vi "enumerateStaticDependencies.vi"(8 "error in (no error)":errorcluster, 11 "SMO.A":refnum<class "SMO.ErrorInjection.lvclass">) -> (0 "error out":errorcluster, 2 "Static Dependencies":refnum<class "Dependency.lvclass">[](array[class]), 3 "SMO.A out":refnum<class "SMO.ErrorInjection.lvclass">)   [LabVIEW 2021, in "SMO.ErrorInjection.lvclass"]
uses:
  SMO.ErrorInjection.lvclass
  SMO.ErrorInjection.lvclass/SMO.ErrorInjection.ctl
  src/SMO/SMO.lvclass
  src/Dependency/Dependency.lvclass
panel:
  # "For instructions on how to use the JKI State Machine Objects, examples and video tutorials, visit:\nhttp://jki.net/state-machine-objects/\n\nJKI State Machine Objects™\nhttp://jki.net/state-machine-objects/\nCopyright (C) 2005-2015, JKI <info@jki.net>\nALL RIGHTS RESERVED"
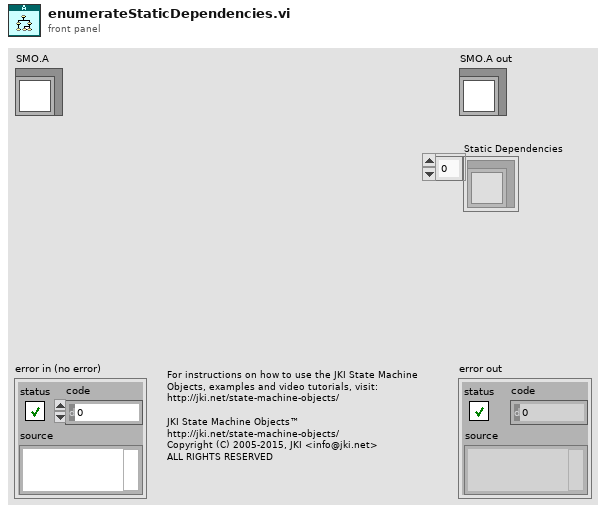
[diagram p1: front panel]
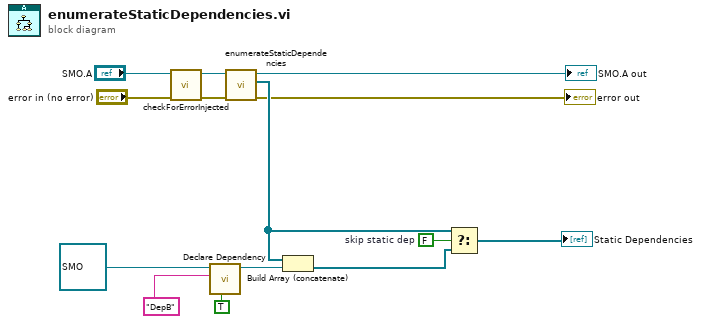
[diagram p0: block diagram]
diagram:
  w14 = FALSE  # skip static dep
  n1 = call "checkForErrorInjected.vi"("error in (no error)"="error in (no error)", "SMO.ErrorInjection in"="SMO.A") -> ("error out"=w9:errorcluster, "SMO.ErrorInjection dup"=w7:refnum<class "SMO.ErrorInjection.lvclass">)  [unwired: 8 in]
  n2 = call "Declare Dependency.vi"("Shared Resource (F)"=TRUE, "Name"="DepB", "Type"=refnum<class "SMO.lvclass"> refnum ("smo.lvlib:SMO.lvclass")) -> ("Dependency out"=w3:refnum<class "Dependency.lvclass">)  [unwired: 7 in, 1 out]
  n3 = call-parent "enumerateStaticDependencies.vi"("error in (no error)"=w9, "SMO"=w7) -> ("error out"=→"error out":errorcluster, "Static Dependencies"=w12:refnum<class "Dependency.lvclass">[], "SMO out"=→"SMO.A out":refnum<class "SMO.ErrorInjection.lvclass">)  [unwired: 7 in]
  n4 = Build Array (concatenate)(w12, w3) -> (w13:refnum<class "Dependency.lvclass">[])
  n5 = Select(t=w12, s=w14, f=w13) -> (s? t:f=→"Static Dependencies":refnum<class "Dependency.lvclass">[])
